vi "Send Data Generator.vi"(7 "Message Priority (Normal)":T2=enum."Normal", 8 "error in (no error)":errorcluster, 9 "Initialization Values":T1={"InitializationParams"={"CurrentPartNumber"="a", "MeasurementData"=[{"MeasurementID"=1, "MeasureEnable"=TRUE, "MeasurementPass"=TRUE, "LimitSets"=[{"LimitSetId"=1, "Limits"=[1.5, 2.2]}]}, {"MeasurementID"=2, "MeasureEnable"=TRUE, "MeasurementPass"=TRUE, "LimitSets"=[{"LimitSetId"=1, "Limits"=[1.8, 2.5]}]}, {"MeasurementID"=3, "MeasureEnable"=TRUE, "MeasurementPass"=TRUE, "LimitSets"=[{"LimitSetId"=1, "Limits"=[2.3, 3.2]}]}, {"MeasurementID"=4, "MeasureEnable"=TRUE, "MeasurementPass"=TRUE, "LimitSets"=[{"LimitSetId"=1, "Limits"=[1.6, 2.4]}]}, {"MeasurementID"=5, "MeasureEnable"=TRUE, "MeasurementPass"=TRUE, "LimitSets"=[{"LimitSetId"=1, "Limits"=[2.5, 3.2]}]}]}}, 10 "I":u32, 11 "Message Enqueuer":refnum<class "Message Enqueuer.lvclass">) -> (0 "error out":errorcluster, 3 "Message Enqueuer out":refnum<class "Message Enqueuer.lvclass">)   [LabVIEW 2015, in "Data Generator Msg.lvclass"]
doc: "This VI sends the message to an actor."
uses:
  Data Generator Msg.lvclass
  <vilib>/ActorFramework/Message Enqueuer/Message Enqueuer.lvclass
  <vilib>/ActorFramework/Message Enqueuer/Message Priority.ctl
  Data Generator Msg.lvclass/Data Generator Msg.ctl
  <vilib>/ActorFramework/Message Enqueuer/Message Enqueuer.lvclass/Message Enqueuer.ctl
  <vilib>/ActorFramework/Message Priority Queue/Priority Enqueue.vi
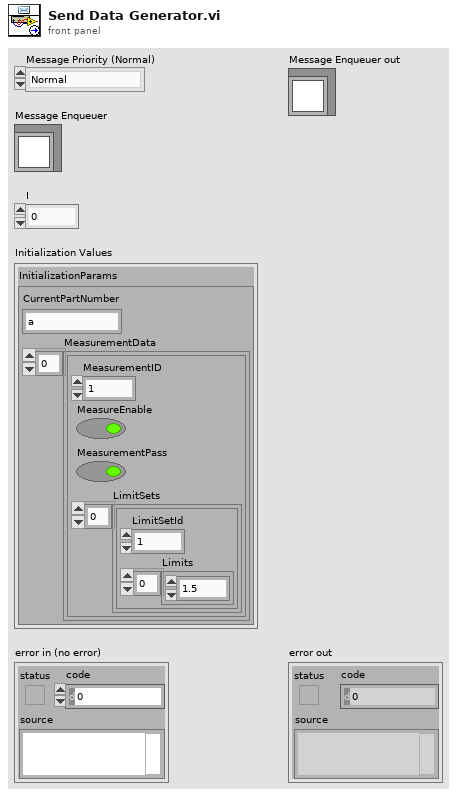
[diagram p1: front panel]
types:
  T1 = cluster{"InitializationParams":cluster{"CurrentPartNumber":string, "MeasurementData":cluster{"MeasurementID":i32, "MeasureEnable":bool, "MeasurementPass":bool, "LimitSets":cluster{"LimitSetId":i32, "Limits":dbl[]}[]}[]}}
  T2 = typedef "Actor Framework.lvlib/Message Enqueuer.lvclass/Message Priority.ctl" = enum16{"Low", "Normal", "High"}
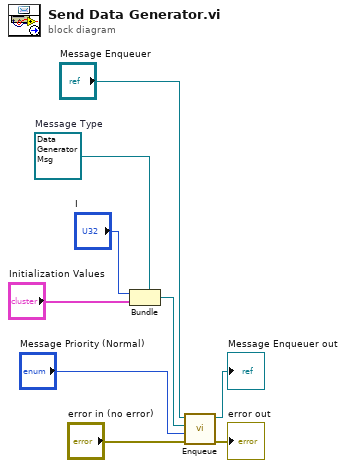
[diagram p0: block diagram]
diagram:
  w6 = refnum<class "Data Generator Msg.lvclass"> refnum  # Message Type
  n1 = Bundle(cluster=w6, "I", "Initialization Values") -> (w5:refnum<class "Data Generator Msg.lvclass">)
  n2 = call <vilib>:"Enqueue.vi"("error in (no error)"="error in (no error)", "Message Priority (Normal)"="Message Priority (Normal)", "Message"=w5, "Message Enqueuer in"="Message Enqueuer") -> ("error out"=→"error out":errorcluster, "Message Enqueuer out"=→"Message Enqueuer out":refnum<class "Message Enqueuer.lvclass">)  [unwired: 6 in]
